vi "obstest.vi"(11 "vehicle width":dbl=2.0 format="%#_13g") -> (0 "lane num":i32, 3 "out":dbl)   [LabVIEW 2015]
uses:
  G_PATH.vi
  G_VEH.vi
  G_SEN.vi
  G_NAV.vi
panel:
  out "element 2":dbl
  out "element":dbl
  out "dy":dbl
  out "path":dbl[](array[numeric])
  out "y":dbl[](array[numeric])
  out "x":dbl[](array[numeric])
  out "y_obs":dbl[](array[numeric])
  out "x_obs":dbl[](array[numeric])
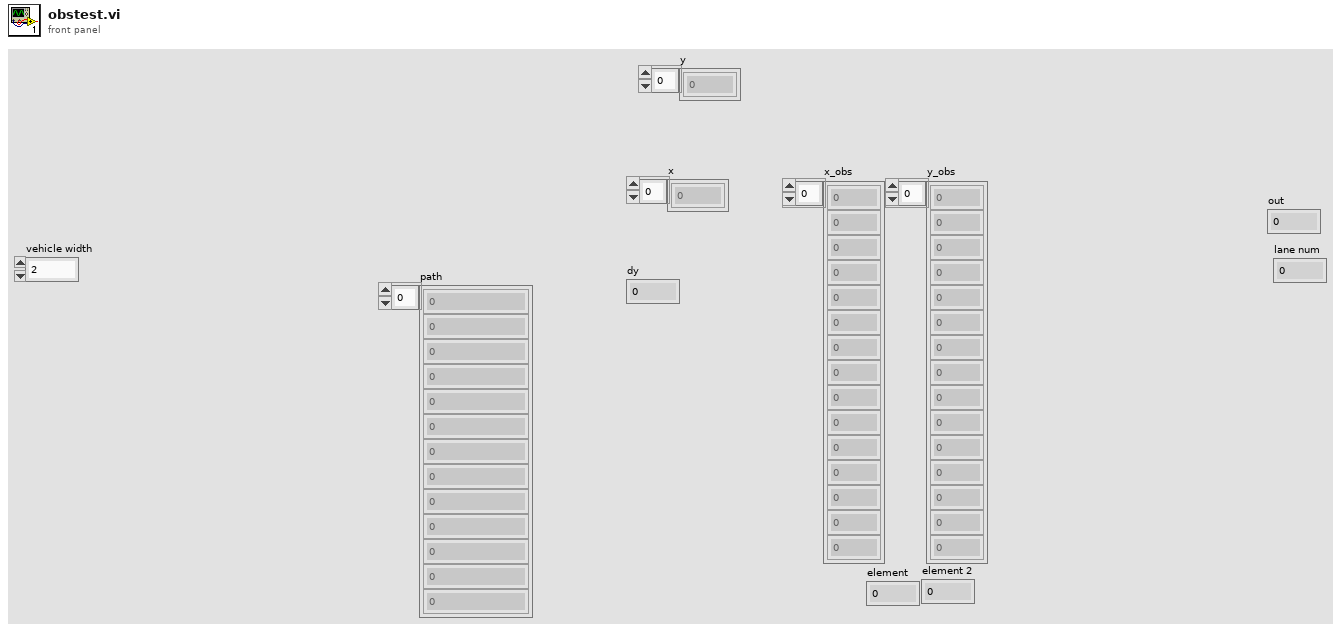
[diagram p1: front panel]
types:
  T1 = cluster{"idx":i32, "x":dbl, "y":dbl, "h":dbl, "x_path":dbl}
  T2 = cluster{"GPSTime":dbl, "attitude[2]":dbl, "lcc[0]":dbl, "lcc[1]":dbl, "heading_GPS":dbl}
  T3 = cluster{"Real Matrix Element":i32, "Real Matrix Element":dbl, "Real Matrix Element":dbl}[]
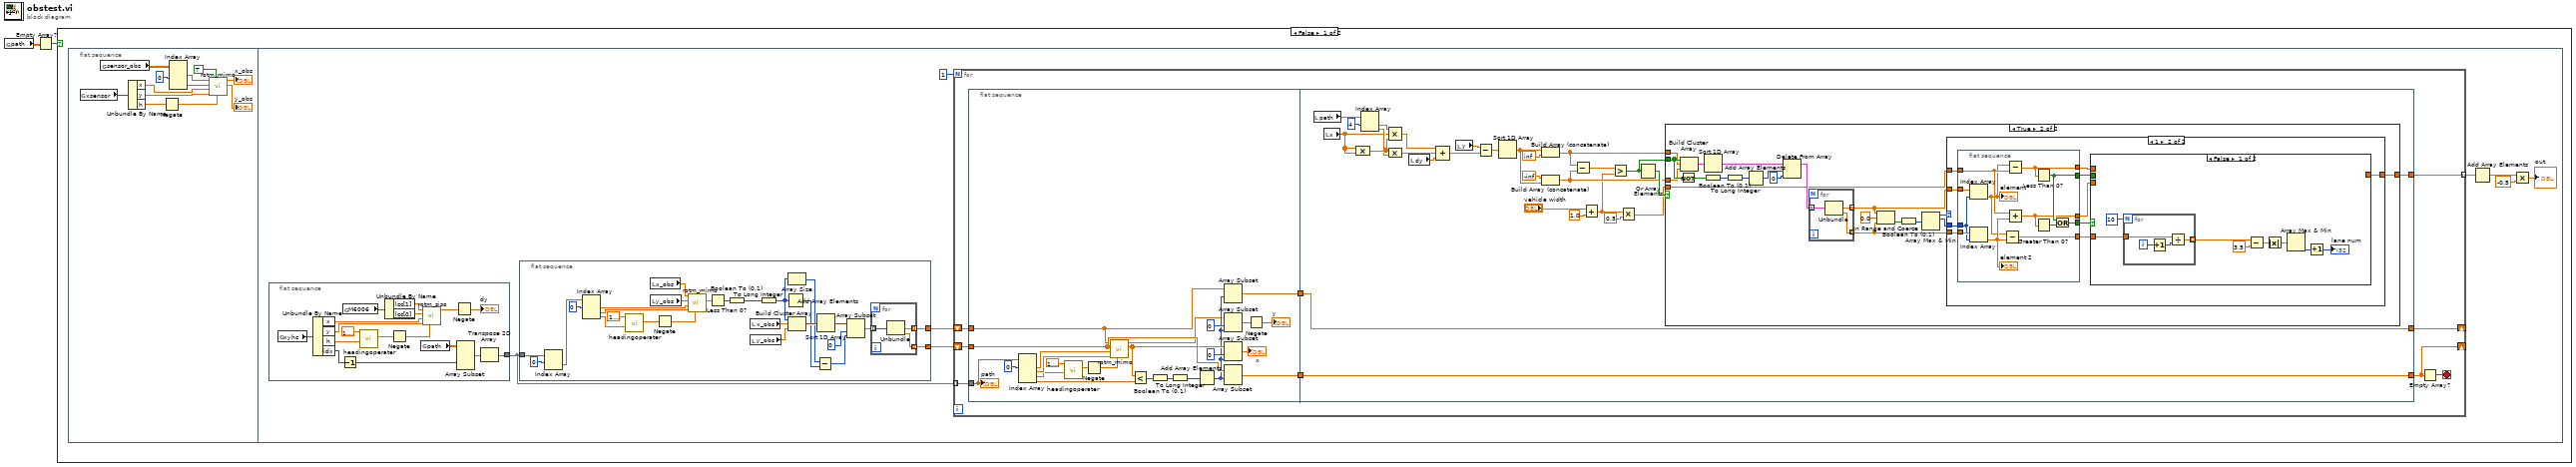
[diagram p0: block diagram]
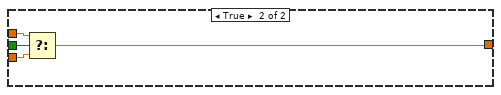
[diagram p4: hidden frame]
diagram:
  n1 = global read "G_PATH.vi" "path"() -> (w2:dbl[][])
  n2 = Empty Array?(array=w2) -> (empty?=w1:bool)
  n3 = case shown="False" w1 {
    frame False {
      n4 = flat-sequence {
        frame #0 {
          n5 = global read "G_VEH.vi" "xsensor"() -> (w8:T1)
          n6 = global read "G_SEN.vi" "sensor_obs"() -> (w7:dbl[][])
          n7 = Unbundle By Name(w8) -> ("x"=w10:dbl, "y"=w11:dbl, "h"=w9:dbl)
          n8 = Negate(x=w9) -> (-x=w12:dbl)
          n9 = Index Array(array=w7, index (col) #1=0 ("disabled index (col)")) -> (element #1=w6:dbl[], element #2=w5:dbl[])  [unwired: 3 in]
          n10 = call "rotm_mimo.vi"("angle[rad]"=w12, "reverse"=TRUE, "y0"=w11, "x0"=w10, "y"=w5, "x"=w6) -> ("Y"=→"y_obs":dbl[], "X"=→"x_obs":dbl[])  [unwired: 2 in, 2 out]
        }
        frame #1 {
          n11 = flat-sequence {
            tunnel: [w64] -> w21
            frame #0 {
              n12 = global read "G_VEH.vi" "xyhc"() -> (w67:T1)
              n13 = Unbundle By Name(w67) -> ("x"=w60:dbl, "y"=w59:dbl, "h"=w56:dbl, "idx"=w68:i32)
              n14 = Decrement(x=w68) -> (x-1=w69:i32)
              n15 = global read "G_NAV.vi" "M6006"() -> (w63:T2)
              n16 = call "headingoperater.vi"("h1"=w56, "h2"=1.5707963267948966) -> ("h2-h1"=w57:dbl)  [unwired: 8 in, 1 out]
              n17 = Unbundle By Name(w63) -> ("lcc[1]"=w62:dbl, "lcc[0]"=w61:dbl)
              n18 = Negate(x=w57) -> (-x=w55:dbl)
              n19 = global read "G_PATH.vi" "path"() -> (w66:dbl[][])
              n20 = call "rotm_siso.vi"("angle[rad]"=w55, "y0"=w59, "x0"=w60, "y"=w61, "x"=w62) -> ("x'"=w54:dbl)  [unwired: 5 in, 1 out]
              n21 = Negate(x=w54) -> (-x=→"dy":dbl)
              n22 = Array Subset(array=w66, index (col)=w69) -> (w65:dbl[][])  [unwired: 3 in]
              n23 = Transpose 2D Array(2D array=w65) -> (transposed array=w64:dbl[][])
            }
          }
          n24 = flat-sequence {
            tunnel: w21 -> [w49]
            tunnel: [w24] -> w20
            tunnel: [w23] -> w19
            frame #0 {
              n25 = Index Array(array=w49, index (row)=0) -> (element=w40:dbl[])  [unwired: 1 in]
              n26 = Index Array(array=w40, index #1=0 ("index")) -> (element #1=w42:dbl, element #2=w43:dbl, element #3=w45:dbl)  [unwired: 2 in]
              n27 = call "headingoperater.vi"("h1"=w45, "h2"=1.5707963267948966) -> ("h2-h1"=w46:dbl)  [unwired: 8 in, 1 out]
              n28 = local read "x_obs"() -> (w38:dbl[])
              n29 = local read "y_obs"() -> (w37:dbl[])
              n30 = Negate(x=w46) -> (-x=w47:dbl)
              n31 = call "rotm_mimo.vi"("angle[rad]"=w47, "y0"=w43, "x0"=w42, "y"=w37, "x"=w38) -> ("Y"=w39:dbl[])  [unwired: 3 in, 3 out]
              n32 = Less Than 0?(x=w39) -> (x < 0?=w33:bool[])
              n33 = Boolean To (0,1)(Boolean=w33) -> (0, 1=w32:i16[])
              n34 = local read "x_obs"() -> (w36:dbl[])
              n35 = local read "y_obs"() -> (w35:dbl[])
              n36 = To Long Integer(number=w32) -> (32bit integer=w29:i32[])
              n37 = Add Array Elements(numeric array=w29) -> (sum=w30:i32)
              n38 = Array Size(array=w29) -> (size(s)=w31:i32)
              n39 = Build Cluster Array(w29, w36, w35) -> (w34:T3)
              n40 = Subtract(x=w31, y=w30) -> (x-y=w27:i32)
              n41 = Sort 1D Array(array=w34) -> (sorted array=w28:T3)
              n42 = Array Subset(array=w28, index=0, length=w27) -> (w25:T3)
              n43 = for {
                tunnel: w25 -> [w52] mode=indexing
                tunnel: [w51] -> w24 mode=indexing
                tunnel: [w50] -> w23 mode=indexing
                n44 = Unbundle(w52) -> ("Real Matrix Element"=w51:dbl, "Real Matrix Element"=w50:dbl)  [unwired: 1 out]
              }
            }
          }
          n45 = for {
            N: 1 -> [_]
            tunnel: w21 -> [w78] mode=indexing
            shift-right: [w75] -> _
            shift-left: w20 -> [w76]
            shift-right: [w71] -> _
            shift-left: w19 -> [w77]
            tunnel: [w70] -> w18 mode=indexing
            stop <- w72 stop-if-true
            n46 = flat-sequence {
              tunnel: w78 -> [w102]
              tunnel: w77 -> [w90]
              tunnel: w76 -> [w88]
              tunnel: [w89] -> w74
              tunnel: [w87] -> w73
              tunnel: [w129] -> w75
              tunnel: [w130] -> w71
              tunnel: w74 -> [w130]
              tunnel: w73 -> [w129]
              tunnel: [w103] -> w70
              frame #0 {
                n47 = Index Array(array=w102, index #1=0 ("index")) -> (element #1=w100:dbl, element #2=w99:dbl, element #3=w97:dbl, element #4=w94:dbl)  [unwired: 3 in]
                n48 = call "headingoperater.vi"("h1"=w97, "h2"=1.5707963267948966) -> ("h2-h1"=w96:dbl)  [unwired: 8 in, 1 out]
                n49 = Negate(x=w96) -> (-x=w95:dbl)
                n50 = call "rotm_mimo.vi"("angle[rad]"=w95, "y0"=w99, "x0"=w100, "y"=w90, "x"=w88) -> ("Y"=w85:dbl[], "X"=w82:dbl[])  [unwired: 3 in, 2 out]
                n51 = Less?(x=w85, y=w94) -> (x < y?=w92:bool[])
                n52 = Boolean To (0,1)(Boolean=w92) -> (0, 1=w93:i16[])
                n53 = To Long Integer(number=w93) -> (32bit integer=w91:i32[])
                n54 = Add Array Elements(numeric array=w91) -> (sum=w83:i32)
                n55 = Array Subset(array=w88, index=w83) -> (w87:dbl[])  [unwired: 1 in]
                n56 = Array Subset(array=w82, index=0, length=w83) -> (w81:dbl[])
                n57 = Array Subset(array=w85, index=0, length=w83) -> (→"x":dbl[])
                n58 = Array Subset(array=w90, index=w83) -> (w89:dbl[])  [unwired: 1 in]
                n59 = Negate(x=w81) -> (-x=→"y":dbl[])
                "path" <- w102
              }
              frame #1 {
                n60 = local read "path"() -> (w128:dbl[])
                n61 = local read "x"() -> (w117:dbl[])
                n62 = Compound Arithmetic op=MULTIPLY(w117, w117) -> (w125:dbl[])
                n63 = Index Array(array=w128, index #1=4 ("index")) -> (element #1=w126:dbl, element #2=w124:dbl)  [unwired: 1 in]
                n64 = Compound Arithmetic op=MULTIPLY(w126, w117, w125) -> (w123:dbl[])
                n65 = Compound Arithmetic op=MULTIPLY(w125, w124) -> (w122:dbl[])
                n66 = local read "dy"() -> (w120:dbl)
                n67 = Compound Arithmetic op=ADD(w123, w122, w120) -> (w118:dbl[])
                n68 = local read "y"() -> (w121:dbl[])
                n69 = Subtract(x=w121, y=w118) -> (x-y=w119:dbl[])
                n70 = Sort 1D Array(array=w119) -> (sorted array=w115:dbl[])
                n71 = Build Array (concatenate)(w115, inf) -> (w107:dbl[])
                n72 = Build Array (concatenate)(-inf, w115) -> (w108:dbl[])
                n73 = Subtract(x=w107, y=w108) -> (x-y=w113:dbl[])
                n74 = Add(x="vehicle width", y=1.0) -> (x+y=w106:dbl)
                n75 = Greater?(x=w113, y=w106) -> (0:w109:bool[])
                n76 = Multiply(x=w106, y=0.5) -> (x*y=w104:dbl)
                n77 = Or Array Elements(Boolean array=w109) -> (logical OR=w110:bool)
                n78 = case shown="True" w110 {
                  tunnel: w109 -> [_ w149]
                  tunnel: w108 -> [_ w140]
                  tunnel: w107 -> [_ w141]
                  tunnel: w104 -> [_ w133]
                  tunnel: [_ w132] -> w103
                  frame False {
                  }
                  frame True {
                    n79 = Not(x=w149) -> (.not. x?=w148:bool[])
                    n80 = Build Cluster Array(w149, w141, w140) -> (w150:cluster{bool, dbl, dbl}[])
                    n81 = Boolean To (0,1)(Boolean=w148) -> (0, 1=w147:i16[])
                    n82 = Sort 1D Array(array=w150) -> (sorted array=w145:cluster{bool, dbl, dbl}[])
                    n83 = To Long Integer(number=w147) -> (32bit integer=w146:i32[])
                    n84 = Add Array Elements(numeric array=w146) -> (sum=w144:i32)
                    n85 = Delete From Array(array=w145, length=w144, index=0) -> (array with subset deleted=w142:cluster{bool, dbl, dbl}[])  [unwired: 1 out]
                    n86 = for {
                      tunnel: w142 -> [w191] mode=indexing
                      tunnel: [w190] -> w136 mode=indexing
                      tunnel: [w189] -> w135 mode=indexing
                      n87 = Unbundle(w191) -> (w190:dbl, w189:dbl)  [unwired: 1 out]
                    }
                    n88 = In Range and Coerce(upper limit=w136, x=0.0, lower limit=w135) -> (In Range?=w138:bool[])  [unwired: 1 out]
                    n89 = Boolean To (0,1)(Boolean=w138) -> (0, 1=w137:i16[])
                    n90 = Array Max & Min(array=w137) -> (max value=w131:i16, max index (indices)=w134:i32)  [unwired: 2 out]
                    n91 = case shown="1" w131 {
                      tunnel: w136 -> [_ w160]
                      tunnel: w135 -> [_ w159]
                      tunnel: w134 -> [_ w158]
                      tunnel: w133 -> [_ w157]
                      tunnel: [_ w154] -> w132
                      frame 0, Default {
                      }
                      frame 1 {
                        n92 = flat-sequence {
                          tunnel: w160 -> [w172]
                          tunnel: w159 -> [w171]
                          tunnel: w158 -> [w170]
                          tunnel: w157 -> [w169]
                          tunnel: [w167] -> w156
                          tunnel: [w166] -> w155
                          tunnel: [w165] -> w153
                          tunnel: [w164] -> w152
                          tunnel: [w163] -> w151
                          frame #0 {
                            n93 = Index Array(array=w172, index=w170) -> (element=w161:dbl)
                            "element" <- w161
                            n94 = Index Array(array=w171, index=w170) -> (element=w162:dbl)
                            "element 2" <- w162
                            n95 = Subtract(x=w161, y=w162) -> (x-y=w163:dbl)
                            n96 = Subtract(x=w161, y=w169) -> (x-y=w165:dbl)
                            n97 = Add(x=w169, y=w162) -> (x+y=w164:dbl)
                            n98 = Less Than 0?(x=w165) -> (x < 0?=w166:bool)
                            n99 = Greater Than 0?(x=w164) -> (x > 0?=w168:bool)
                            n100 = Or(x=w166, y=w168) -> (x .or. y?=w167:bool)
                          }
                        }
                        n101 = case shown="False" w156 {
                          tunnel: w155 -> [_ w188]
                          tunnel: w153 -> [_ w187]
                          tunnel: w152 -> [_ w186]
                          tunnel: [_ w185] -> w154
                          tunnel: w151 -> [w180 _]
                          frame False {
                            n102 = for {
                              N: 10 -> [_]
                              tunnel: w180 -> [w182]
                              tunnel: [w181] -> w178 mode=indexing
                              i -> [w184]
                              n103 = Increment(x=w184) -> (x+1=w183:i32)
                              n104 = Divide(x=w182, y=w183) -> (x/y=w181:dbl)
                            }
                            n105 = Subtract(x=w178, y=3.5) -> (x-y=w176:dbl[])
                            n106 = Absolute Value(x=w176) -> (abs(x)=w175:dbl[])
                            n107 = Array Max & Min(array=w175) -> (min index (indices)=w174:i32)  [unwired: 3 out]
                            n108 = Increment(x=w174) -> (x+1=→"lane num":i32)
                          }
                          frame True {
                            n109 = Select(t=w187, s=w188, f=w186) -> (s? t:f=w185:dbl)
                          }
                        }
                      }
                    }
                  }
                }
              }
            }
            n110 = Empty Array?(array=w71) -> (empty?=w72:bool)
          }
          n111 = Add Array Elements(numeric array=w18) -> (sum=w17:dbl)
          n112 = Multiply(x=w17, y=-0.5) -> (x*y=→"out":dbl)
        }
      }
    }
    frame True {
    }
  }
